vi "PIO.Read U32 Array.vi"(8 "error in (no error)":errorcluster, 9 "count":u32, 10 "offset":u32 format="%.0x", 11 "GE 5565PIORC in":refnum<class "GE 5565PIORC.lvclass">) -> (0 "error out":errorcluster, 2 "values":u32[](array[numeric]), 3 "GE 5565PIORC out":refnum<class "GE 5565PIORC.lvclass">)   [LabVIEW 2016, in "GE 5565PIORC.lvclass"]
uses:
  GE 5565PIORC.lvclass
  GE 5565PIORC.lvclass/GE 5565PIORC.ctl
  <vilib>/Instr/_visa.llb/VISA Register Access Address Space.ctl
  Change Endianness (U32).vi
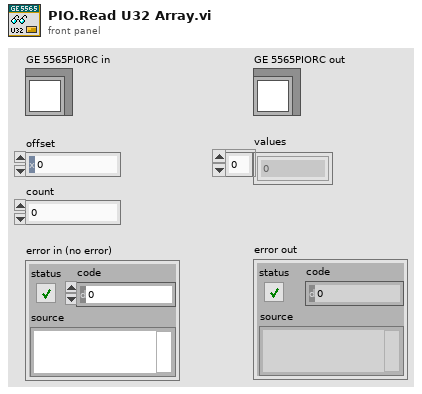
[diagram p1: front panel]
types:
  T1 = typedef "VISA Register Access Address Space.ctl" = u16
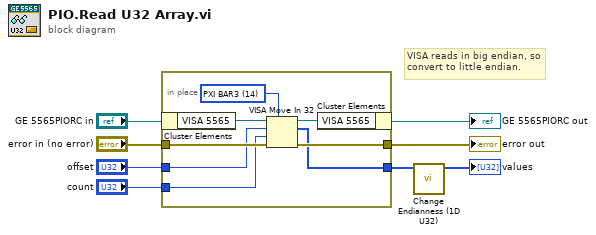
[diagram p0: block diagram]
diagram:
  # "VISA reads in big endian, so convert to little endian."
  n1 = in-place {
    in-place-border: "error in (no error)" -> [w16]
    in-place-border: [w15] -> w7
    in-place-border: "offset" -> [w11]
    in-place-border: [w10] -> w2
    in-place-border: "count" -> [w9]
    w12 = T1 14 items=["VXI/VME A16"=1, "VXI/VME A24"=2, "VXI/VME A32"=3, "VXI/VME A64"=4, "PXI Memory Allocations"=9, "PXI Configuration"=10, "PXI BAR0"=11, "PXI BAR1"=12, "PXI BAR2"=13, "PXI BAR3"=14, "PXI BAR4"=15, "PXI BAR5"=16] ("Address Space")
    n2 = in-place-cluster #1("GE 5565PIORC in") -> ("VISA 5565"=w14:refnum<visa-resource-name>)
    n3 = VISA Move In 32(7:w12, 8:w16, 9:w9, 10:w11, 11:w14) -> (0:w15:errorcluster, 2:w10:u32[], 3:w13:refnum<visa-resource-name>)
    n4 = in-place-cluster #1("VISA 5565"=w13) -> (→"GE 5565PIORC out":refnum<class "GE 5565PIORC.lvclass">)
  }
  "error out" <- w7
  n5 = call "Change Endianness (1D U32).vi"("array in"=w2) -> ("byte-reversed array out"=→"values":u32[])  [unwired: 10 in]
